vi "Get pedal status.vi"(7 "timeout in ms (-1)":i32=-1, 8 "Error Queue":refnum<queue>, 10 "Update Motors Notifier":refnum<notifier>, 11 "CAN Session In":T1=refnum) -> (0 "Exit?":bool, 2 "\"Pedals\" Status":T2 {"Acceleration pedal" scale=0.0..100.0 scale format="%#_6f%%"; "Break pedal" scale=0.0..100.0 scale format="%#_6f%%"}, 3 "Last Pedals Update":u32)   [LabVIEW 2016]
uses:
  RT/Pedals Status.ctl
  Program Files (x86)/National Instruments/LabVIEW 2016/examples/robotics/EPOS2 CANOpen Driver/Low Level VIs/Typedefs/CAN Refnum.ctl
  Program Files (x86)/National Instruments/LabVIEW 2016/examples/robotics/EPOS2 CANOpen Driver/Low Level VIs/Typedefs/CAN Session Pointer.ctl
  Program Files (x86)/National Instruments/LabVIEW 2016/examples/robotics/EPOS2 CANOpen Driver/Low Level VIs/Typedefs/CAN Communication References.ctl
  Program Files (x86)/National Instruments/LabVIEW 2016/examples/robotics/EPOS2 CANOpen Driver/Low Level VIs/Typedefs/kill process notifier array.ctl
  Program Files (x86)/National Instruments/LabVIEW 2016/examples/robotics/EPOS2 CANOpen Driver/Low Level VIs/Typedefs/Write Queue.ctl
  Program Files (x86)/National Instruments/LabVIEW 2016/examples/robotics/EPOS2 CANOpen Driver/Low Level VIs/Typedefs/FPGA CAN Frame Cluster.ctl
  RT/Read single CAN.vi
  RT/Data to Pedals Status.vi
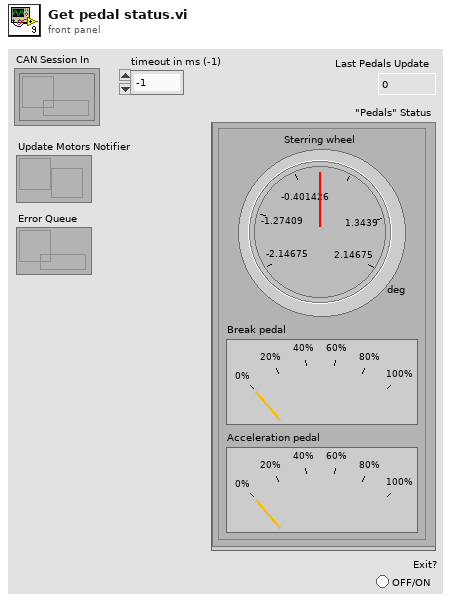
[diagram p1: front panel]
types:
  T1 = typedef "CAN Refnum.ctl" = refnum<k1>
  T2 = typedef "Pedals Status.ctl" = cluster{"Acceleration pedal":dbl, "Break pedal":dbl, "Sterring wheel":dbl[unit]}
  T3 = typedef "FPGA CAN Frame Cluster.ctl" = cluster{"Timestamp":u64, "Identifier":u32, "Type":u8, "InfoA":u8, "InfoB":u8, "DataLength":u8, "Data":u8[]}
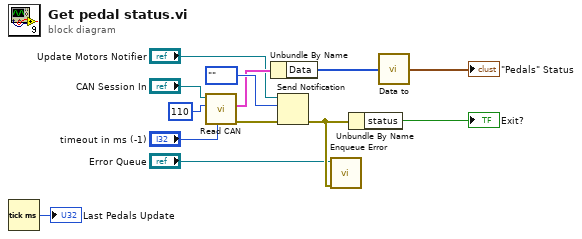
[diagram p0: block diagram]
diagram:
  n1 = Tick Count (ms)() -> (millisecond timer value=→"Last Pedals Update":u32)
  n2 = call-poly "Read CAN.vi"("timeout in ms (-1)"="timeout in ms (-1)", "ID"=110, "CAN Session In"="CAN Session In") -> ("error out"=w12:errorcluster, "CAN Frame Out"=w11:T3)  [unwired: 6 in, 1 out]
  n3 = Unbundle By Name(w11) -> ("Data"=w10:u8[])
  n4 = Send Notification(notification=enum16{""}."", notifier="Update Motors Notifier", error in (no error)=w12) -> (error out=w2:errorcluster)  [unwired: 1 out]
  n5 = call "Enqueue Error.vi"("error in"=w2, "Error Queue"="Error Queue") -> ()  [unwired: 10 in]
  n6 = Unbundle By Name(w2) -> ("status"=→"Exit?":bool)
  n7 = call-poly "Data to.vi"("Data"=w10) -> ("\"Pedals\" Status"=→"\"Pedals\" Status":T2)
